vi "add assembly.vi"(5 "big endian?":bool, 6 "size (bytes)":u32=32, 7 "name":string, 8 "error in":errorcluster, 9 "Type":T1, 10 "instance ID":u32=100, 11 "EthernetIP configuration in":refnum<class "EthernetIP configuration.lvclass">) -> (0 "error out":errorcluster, 3 "EthernetIP configuration out":refnum<class "EthernetIP configuration.lvclass">)   [LabVIEW 2013, in "EthernetIP configuration.lvclass"]
uses:
  EthernetIP configuration.lvclass
  assembly type.ctl
  EthernetIP configuration.lvclass/EthernetIP configuration.ctl
  assembly definition.ctl
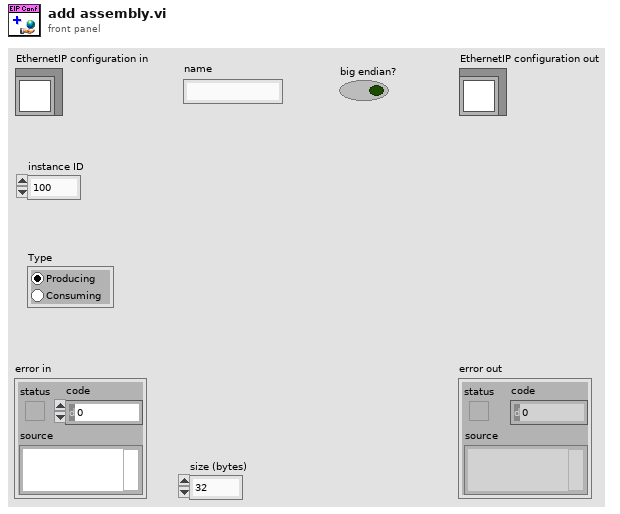
[diagram p1: front panel]
types:
  T1 = typedef "EthernetIP configuration.lvclass/assembly type.ctl" = enum32{"Producing", "Consuming"}
  T2 = typedef "EthernetIP configuration.lvclass/assembly definition.ctl" = cluster{"name":string, "Instance ID":u32, "Type":T1, "Size (bytes)":u32, "big endian?":bool}
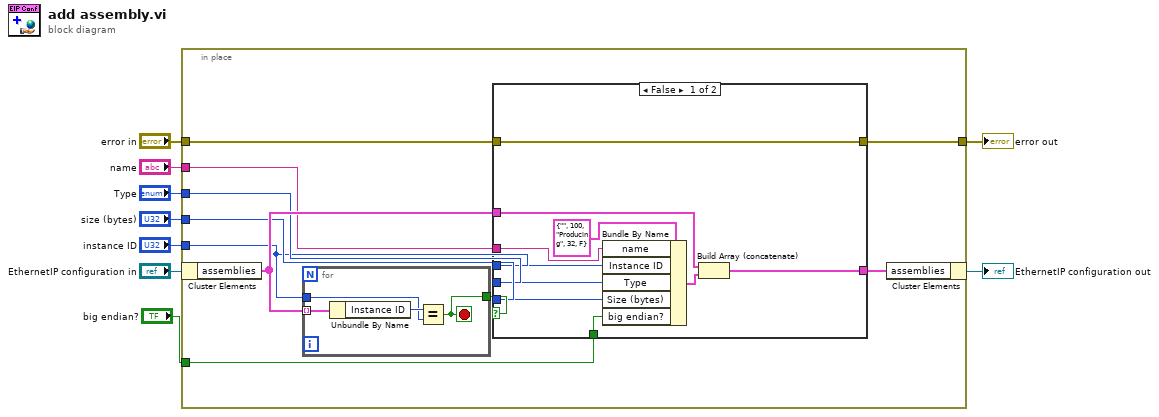
[diagram p0: block diagram]
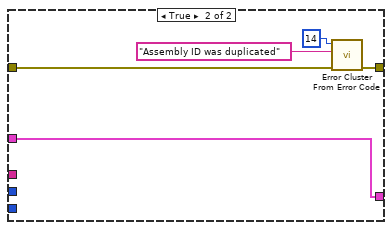
[diagram p2: hidden frame]
diagram:
  n1 = in-place {
    in-place-border: "instance ID" -> [w12]
    in-place-border: "error in" -> [w16]
    in-place-border: [w15] -> w5
    in-place-border: "size (bytes)" -> [w14]
    in-place-border: "Type" -> [w13]
    in-place-border: "name" -> [w11]
    in-place-border: "big endian?" -> [w10]
    n2 = in-place-cluster #1("EthernetIP configuration in") -> ("assemblies"=w17:T2[])
    n3 = for {
      tunnel: w17 -> [w38] mode=indexing
      tunnel: w12 -> [w36]
      tunnel: [w35] -> w19
      stop <- w35 stop-if-true
      n4 = Unbundle By Name(w38) -> ("Instance ID"=w37:u32)
      n5 = Equal?(x=w37, y=w36) -> (x = y?=w35:bool)
    }
    n6 = case shown="False" w19 {
      tunnel: [w27 w34] -> w18
      tunnel: w17 -> [w28 w34]
      tunnel: w16 -> [w29 w31]
      tunnel: [w29 w30] -> w15
      tunnel: w14 -> [w25 _]
      tunnel: w13 -> [w24 _]
      tunnel: w12 -> [w23 _]
      tunnel: w11 -> [w22 _]
      tunnel: w10 -> [w20 _]
      frame False {
        n7 = Bundle By Name(cluster=T2 {"name"="", "Instance ID"=100, "Type"=enum."Producing", "Size (bytes)"=32, "big endian?"=FALSE} ("assembly definition"), "name"=w22, "Instance ID"=w23, "Type"=w24, "Size (bytes)"=w25, "big endian?"=w20) -> (w21:T2)
        n8 = Build Array (concatenate)(w28, w21) -> (w27:T2[])
      }
      frame True {
        n9 = call <vilib>:"Error Cluster From Error Code.vi"("error in (no error)"=w31, "error message (\"\")"="Assembly ID was duplicated" ("error message (\"\")"), "error code (0)"=14) -> ("error out"=w30:errorcluster)  [unwired: 6 in]
      }
    }
    n10 = in-place-cluster #1("assemblies"=w18) -> (→"EthernetIP configuration out":refnum<class "EthernetIP configuration.lvclass">)
  }
  "error out" <- w5
